vi "Delete Empty File.vi"(1 "error in":errorcluster, 2 "Path":path) -> (0 "error out":errorcluster)   [LabVIEW 2010]
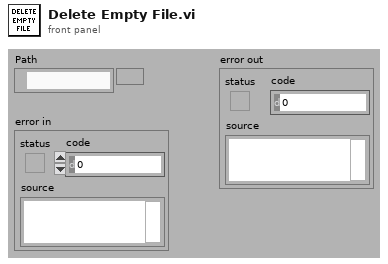
[diagram p1: front panel]
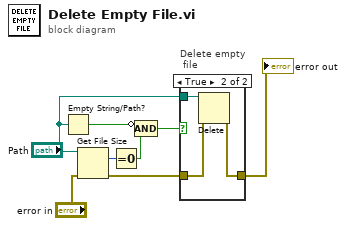
[diagram p0: block diagram]
diagram:
  n1 = Empty String/Path?(string/path="Path") -> (empty?=w6:bool)
  n2 = Get File Size(file="Path", error in="error in") -> (size (in bytes)=w1:i64, 0:w3:errorcluster)  [unwired: 1 out]
  n3 = Equal To 0?(x=w1) -> (x = 0?=w7:bool)
  n4 = Compound Arithmetic op=AND(invert w6, w7) -> (w8:bool)
  n5 = case "Delete empty\n file" shown="True" w8 {
    tunnel: "Path" -> [_ w12]
    tunnel: w3 -> [w9 w11]
    tunnel: [w9 w10] -> w4
    frame False {
    }
    frame True {
      n6 = Delete(path (use dialog)=w12, error in=w11) -> (error out=w10:errorcluster)  [unwired: 3 in, 2 out]
    }
  }
  "error out" <- w4
